vi "读取A1外设配置.vi"(8 "error in (no error)":errorcluster, 11 "MB session in":refnum<class "MB_Master.lvclass">) -> (0 "error out":errorcluster, 2 "外设配置":T1 {"总氮x公式0" items=["0", "1"]; "光谱仪类型" items=["1型", "2型", "3型", "2型氙灯联控"]; "泵阀量" items=["9通"=9, "10通"=10, "12通"=12]; "泵类型" items=["1型", "2型", "sy04型+旋转阀"]}, 3 "MB session out":refnum<class "MB_Master.lvclass">)   [LabVIEW 2016, in "斯坦道总氮.lvlib"]
uses:
  <vilib>/Plasmionique/MB Master/MB_Master/MB_Master.lvclass
  <vilib>/Plasmionique/MB Master/MB_Master_Serial/MB_Master_Serial.lvclass
  C:/Program Files (x86)/National Instruments/LabVIEW 2016/vi.lib/Plasmionique/MB Master/MB_Master/MB_Master.lvclass
  <vilib>/Plasmionique/MB Master/MB Master.lvlib
panel:
  in  "VISA Resource":refnum<visa-resource-name>
  in  "引用选择":enum16{"MB引用", "自建引用"}(ring)
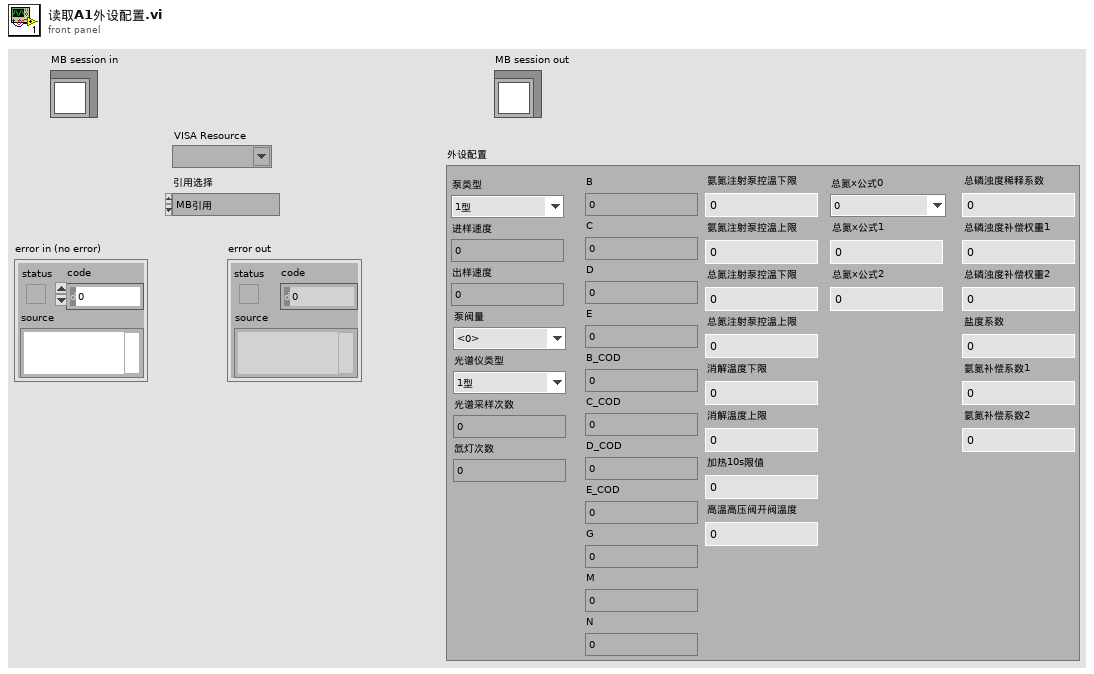
[diagram p1: front panel]
types:
  T1 = typedef "斯坦道总氮.lvlib/V3 A1版外设参数.ctl" = cluster{"泵类型":u8, "进样速度":u32, "出样速度":u32, "泵阀量":u8, "光谱仪类型":u8, "光谱采样次数":u8, "氙灯次数":u8, "B":u16, "C":u16, "D":u16, "E":u16, "B_COD":u16, "C_COD":u16, "D_COD":u16, "E_COD":u16, "G":u16, "M":u16, "N":u16, "氨氮注射泵控温下限":sgl, "氨氮注射泵控温上限":sgl, "总氮注射泵控温下限":sgl, "总氮注射泵控温上限":sgl, "消解温度下限":sgl, "消解温度上限":sgl, "加热10s限值":sgl, "高温高压阀开阀温度":sgl, "总氮x公式0":u8, "总氮x公式1":sgl, "总氮x公式2":sgl, "总磷浊度稀释系数":sgl, "总磷浊度补偿权重1":sgl, "总磷浊度补偿权重2":sgl, "盐度系数":sgl, "氨氮补偿系数1":sgl, "氨氮补偿系数2":sgl}
  T2 = cluster{"baud rate (bps)":u32, "stop bits":u16, "parity":u16, "flow control":u16, "timeout":u32, "retries":i32}
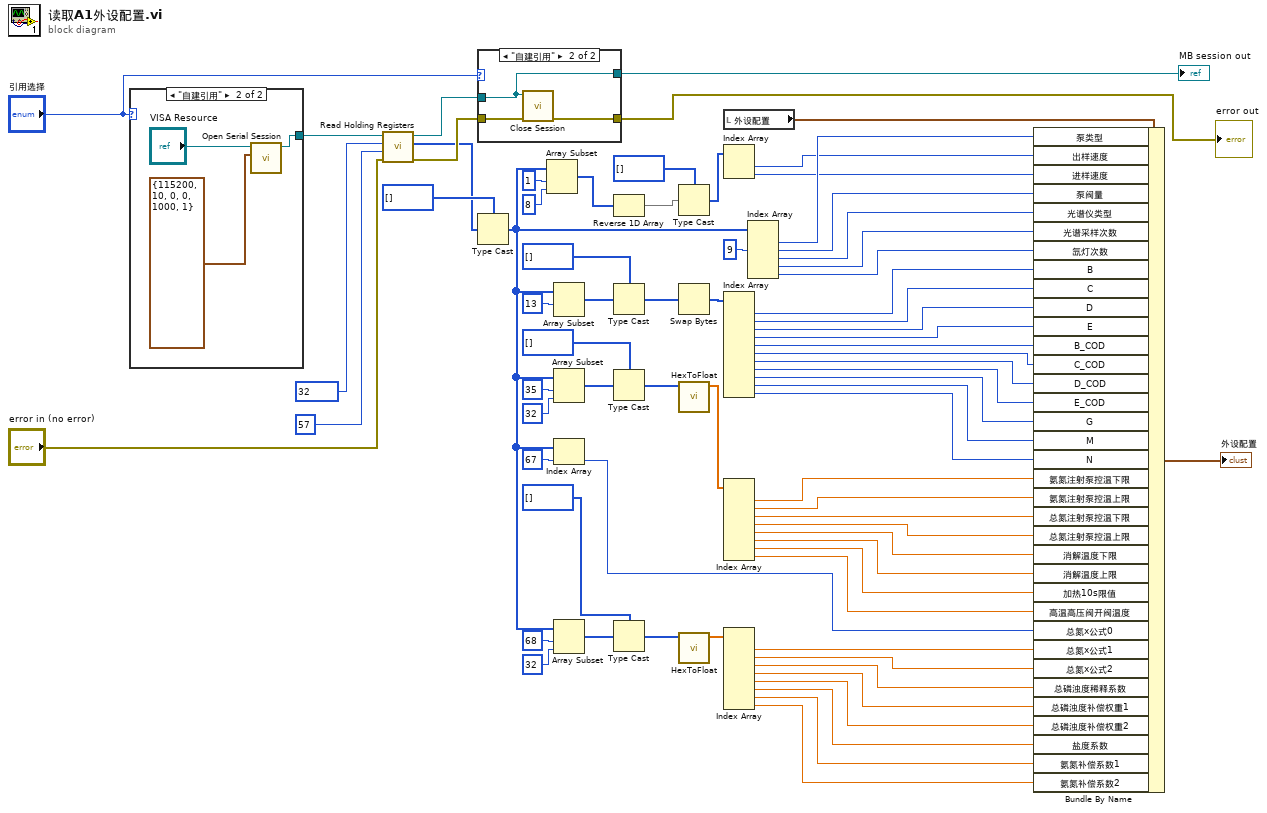
[diagram p0: block diagram]
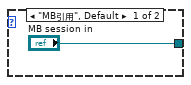
[diagram p3: hidden frame]
diagram:
  n1 = case shown="\"自建引用\"" "引用选择" {
    tunnel: ["MB session in" w78] -> w64
    frame "MB引用", Default {
    }
    frame "自建引用" {
      n2 = call <vilib>:"Open Serial Session.vi"("Serial Config"=T2 {"baud rate (bps)"=115200, "stop bits"=10, "parity"=0, "flow control"=0, "timeout"=1000, "retries"=1}, "VISA Resource"="VISA Resource") -> ("MB_Serial session"=w78:refnum<class "MB_Master_Serial.lvclass">)  [unwired: 8 in, 1 out]
    }
  }
  n3 = call <vilib>:"Read Holding Registers.vi"("error in (no error)"="error in (no error)", "quantity"=u16 57, "starting address"=u16 32, "MB session in"=w64) -> ("error out"=w61:errorcluster, "Registers"=w40:u16[], "MB session out"=w63:refnum<class "MB_Master.lvclass">)  [unwired: 5 in]
  n4 = case shown="\"自建引用\"" "引用选择" {
    tunnel: w63 -> [w79 w81]
    tunnel: w61 -> [w80 w83]
    tunnel: [w80 w82] -> w60
    tunnel: [w79 w81] -> w59
    frame "MB引用", Default {
    }
    frame "自建引用" {
      n5 = call-dynamic "Close Session.vi"("error in (no error)"=w83, "MB session in"=w81) -> ("error out"=w82:errorcluster)  [unwired: 9 in]
    }
  }
  "MB session out" <- w59
  "error out" <- w60
  n6 = Type Cast(type=u8[] [], x=w40) -> (*(type *) &x=w39:u8[])
  n7 = Array Subset(array=w39, index=1 ("索引"), length=8 ("长度")) -> (w68:u8[])
  n8 = Array Subset(array=w39, index=13 ("索引")) -> (w50:u8[])  [unwired: 1 in]
  n9 = Array Subset(array=w39, index=35 ("索引"), length=32 ("长度")) -> (w55:u8[])
  n10 = Index Array(array=w39, index=67 ("索引")) -> (element=w14:u8)
  n11 = Array Subset(array=w39, index=68 ("索引"), length=32 ("长度")) -> (w45:u8[])
  n12 = Reverse 1D Array(array=w68) -> (reversed array=w67:u8[])
  n13 = Type Cast(type=u16[] [], x=w50) -> (*(type *) &x=w49:u16[])
  n14 = Type Cast(type=u16[] [], x=w55) -> (*(type *) &x=w53:u16[])
  n15 = Type Cast(type=u16[] [], x=w45) -> (*(type *) &x=w44:u16[])
  n16 = Type Cast(type=u32[] [], x=w67) -> (*(type *) &x=w65:u32[])
  n17 = Swap Bytes(anything=w49) -> (byte swapped=w48:u16[])
  n18 = call "HexToFloat.vi"("数组"=w53) -> ("FLOAT"=w56:sgl[])  [unwired: 10 in]
  n19 = call "HexToFloat.vi"("数组"=w44) -> ("FLOAT"=w46:sgl[])  [unwired: 10 in]
  n20 = local read "外设配置"() -> (w38:T1)
  n21 = Index Array(array=w65) -> (element #1=w35:u32, element #2=w34:u32)  [unwired: 2 in]
  n22 = Index Array(array=w48) -> (element #1=w32:u16, element #2=w31:u16, element #3=w30:u16, element #4=w29:u16, element #5=w28:u16, element #6=w27:u16, element #7=w26:u16, element #8=w25:u16, element #9=w24:u16, element #10=w23:u16, element #11=w22:u16)  [unwired: 11 in]
  n23 = Index Array(array=w56) -> (element #1=w21:sgl, element #2=w20:sgl, element #3=w19:sgl, element #4=w18:sgl, element #5=w17:sgl, element #6=w16:sgl, element #7=w15:sgl, element #8=w1:sgl)  [unwired: 8 in]
  n24 = Index Array(array=w46) -> (element #1=w13:sgl, element #2=w12:sgl, element #3=w11:sgl, element #4=w10:sgl, element #5=w9:sgl, element #6=w8:sgl, element #7=w7:sgl, element #8=w6:sgl)  [unwired: 8 in]
  n25 = Index Array(array=w39, index #2=9 ("索引")) -> (element #1=w36:u8, element #2=w33:u8, element #3=w4:u8, element #4=w3:u8, element #5=w2:u8)  [unwired: 4 in]
  n26 = Bundle By Name(cluster=w38, "泵类型"=w36, "出样速度"=w35, "进样速度"=w34, "泵阀量"=w33, "光谱仪类型"=w4, "光谱采样次数"=w3, "氙灯次数"=w2, "B"=w32, "C"=w31, "D"=w30, "E"=w29, "B_COD"=w28, "C_COD"=w27, "D_COD"=w26, "E_COD"=w25, "G"=w24, "M"=w23, "N"=w22, "氨氮注射泵控温下限"=w21, "氨氮注射泵控温上限"=w20, "总氮注射泵控温下限"=w19, "总氮注射泵控温上限"=w18, "消解温度下限"=w17, "消解温度上限"=w16, "加热10s限值"=w15, "高温高压阀开阀温度"=w1, "总氮x公式0"=w14, "总氮x公式1"=w13, "总氮x公式2"=w12, "总磷浊度稀释系数"=w11, "总磷浊度补偿权重1"=w10, "总磷浊度补偿权重2"=w9, "盐度系数"=w8, "氨氮补偿系数1"=w7, "氨氮补偿系数2"=w6) -> (→"外设配置":T1)
